vi "Windows Dialog Box DLL.vi"(4 "Icon (None)":T2(ring), 5 "Beep? (F)":bool, 6 "Window Buttons (OK)":T3(ring), 7 "Modality (System)":enum16{"Application", "System", "Task"}(ring)=enum."System", 8 "error in (no error)":errorcluster, 10 "Message":string, 11 "Title":string) -> (0 "error out":errorcluster, 3 "Button Pressed":T1(ring))   [LabVIEW 2011]
doc: "This VI calls the Windows functions MessageBox and MessageBeep to display a message dialog box and, optionally, play a sound effect. These functions are in the Windows DLL called USER.EXE, which is located in the windows\\system directory. If your computer is not equipped with a sound driver, a short \"beep\" will be played through the PC's speaker.\n\nVarious combinations of dialog boxes are possible. The buttons input selects which buttons are displayed in the dialog box, the icon input determines the icon, if any, and the modality box determines whether the dialog box is system, application, or task modal.\n\nIf sounds are enabled, the icon option determines the sound effect played, as defined in the Sounds section of Windows' Control Panel.\n\nThe DLL functions called are:\n\nint MessageBox ( hWndParent, lpText, lpCaption, wType )\nvoid MessageBeep ( wType )\n\nFunction definitions are from:\nMicrosoft Windows Programmer's Reference\nCopyright 1990 Microsoft Corporation.\n\n-------------\nBrian Hoover aka Hooovahh"
uses:
  User32.dll
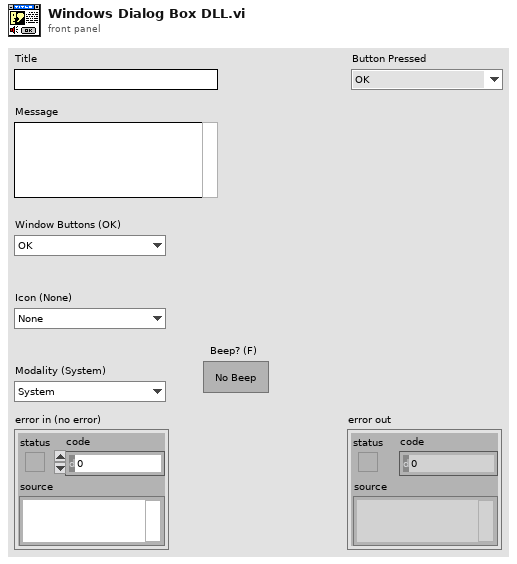
[diagram p1: front panel]
types:
  T1 = enum16{"OK", "Cancel", "Abort", "Retry", "Ignore", "Yes", "No"}
  T2 = enum16{"None", "Stop", "Question Mark", "Exclamation", "Information"}
  T3 = enum16{"OK", "OK/Cancel", "Abort/Retry/Ignore", "Yes/No/Cancel", "Yes/No", "Retry Cancel"}
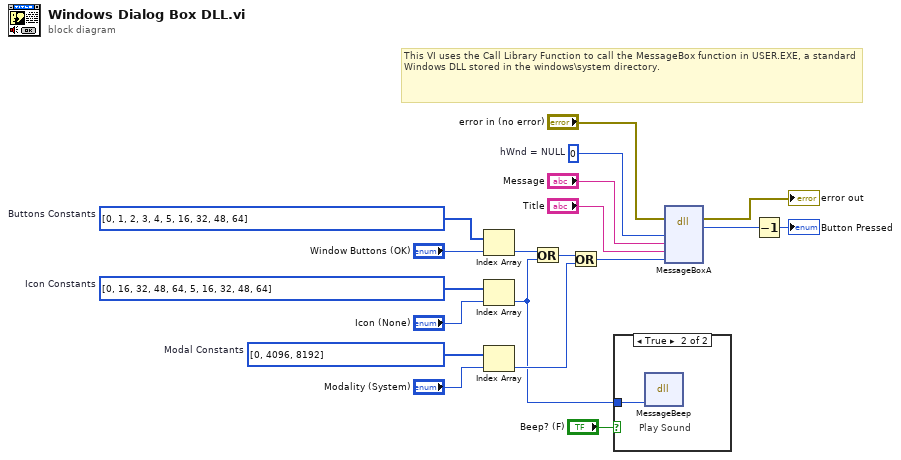
[diagram p0: block diagram]
diagram:
  w11 = i32[] [0, 16, 32, 48, 64, 5, 16, 32, 48, 64]  # Icon Constants
  w14 = i32[] [0, 4096, 8192]  # Modal Constants
  w12 = i32[] [0, 1, 2, 3, 4, 5, 16, 32, 48, 64]  # Buttons Constants
  w18 = u32 0  # hWnd = NULL
  # "This VI uses the Call Library Function to call the MessageBox function in USER.EXE, a standard Windows DLL stored in the windows\\system directory."
  n1 = Index Array(array=w12, index="Window Buttons (OK)") -> (element=w10:i32)
  n2 = Index Array(array=w11, index="Icon (None)") -> (element=w7:i32)
  n3 = Index Array(array=w14, index="Modality (System)") -> (element=w9:i32)
  n4 = Or(x=w10, y=w7) -> (x .or. y?=w8:i32)
  n5 = Or(x=w8, y=w9) -> (x .or. y?=w13:i32)
  n6 = case shown="True" "Beep? (F)" {
    tunnel: w7 -> [_ w20]
    frame False {
      # "Do not play sound effects."
    }
    frame True {
      # "Play Sound"
      n7 = dll-call lib="USER32.DLL" fn="MessageBeep"("wType"=w20) -> ()  [unwired: 4 in, 3 out]
    }
  }
  n8 = dll-call lib="USER32.DLL" fn="MessageBoxA" label="MessageBox"(error in="error in (no error)", "hWndParent"=w18, "lpText"="Message", "lpCaption"="Title", "wType"=w13) -> (error out=→"error out":errorcluster, w15:i32)  [unwired: 6 in, 1 out]
  n9 = Decrement(x=w15) -> (x-1=→"Button Pressed":i32)
